vi "Configure BUS Source.vi"   [LabVIEW 2009, in "Tektronix DPO MSO 2000 4000 Series.lvlib"]
doc: "The polymorphic VI includes VIs that configures I2C bus, SPI bus and CAN bus settings for an oscilloscope."
uses:
  <instrlib>/Tektronix DPO MSO 2000 4000 Series/Tektronix DPO MSO 2000 4000 Series.lvlib
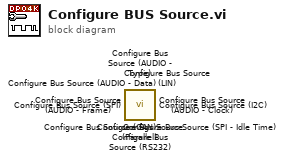
[diagram p0: block diagram]
diagram:
  n1 = call <instrlib>:"Configure Bus Source (Parallel).vi"() -> ()  [unwired: 14 in, 2 out]
  n2 = call <instrlib>:"Configure Bus Source (LIN).vi"() -> ()  [unwired: 14 in, 2 out]
  n3 = call <instrlib>:"Configure Bus Source (AUDIO - Frame).vi"() -> ()  [unwired: 14 in, 2 out]
  n4 = call <instrlib>:"Configure Bus Source (AUDIO - Clock).vi"() -> ()  [unwired: 14 in, 2 out]
  n5 = call <instrlib>:"Configure Bus Source (AUDIO - Data).vi"() -> ()  [unwired: 14 in, 2 out]
  n6 = call <instrlib>:"Configure Bus Source (AUDIO - Type).vi"() -> ()  [unwired: 14 in, 2 out]
  n7 = call <instrlib>:"Configure Bus Source (SPI - Idle Time).vi"() -> ()  [unwired: 14 in, 2 out]
  n8 = call <instrlib>:"Configure Bus Source (RS232).vi"() -> ()  [unwired: 14 in, 2 out]
  n9 = call <instrlib>:"Configure Bus Source (SPI).vi"() -> ()  [unwired: 14 in, 2 out]
  n10 = call <instrlib>:"Configure Bus Source (I2C).vi"() -> ()  [unwired: 14 in, 2 out]
  n11 = call <instrlib>:"Configure Bus Source (CAN).vi"() -> ()  [unwired: 14 in, 2 out]
